vi "Memory.Pointer.Read.vi"(8 "error in (no error)":errorcluster, 9 "offset (0)":u64 format="%d bytes", 10 "length (-1: all)":i64=-1 format="%d bytes", 11 "Pointer in":refnum<class "Memory.Pointer.lvclass">) -> (0 "error out":errorcluster, 2 "data":string, 3 "Pointer out":refnum<class "Memory.Pointer.lvclass">)   [LabVIEW 2016, in "LabVIEW Memory Manager.lvlib" / "Memory.Pointer.lvclass"]
uses:
  Memory.Pointer.lvclass
  Memory.Pointer.lvclass/Memory.Pointer.ctl
  Accessors/Memory.Pointer.Get Address.vi
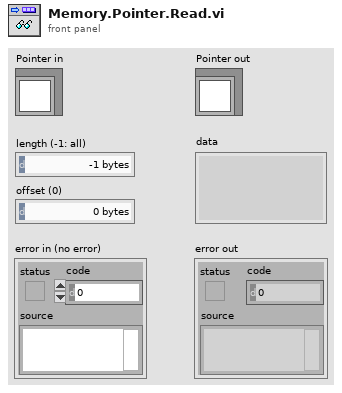
[diagram p1: front panel]
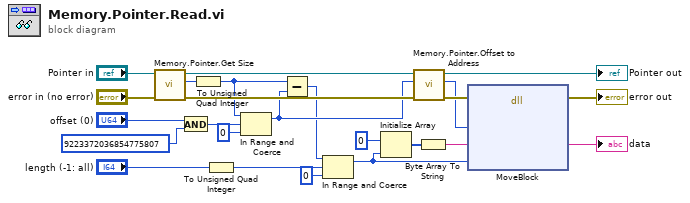
[diagram p0: block diagram]
diagram:
  n1 = call "Memory.Pointer.Get Size.vi"("error in (no error)"="error in (no error)", "Pointer in"="Pointer in") -> ("error out"=w18:errorcluster, "size"=w9:i64, "Pointer out"=w19:refnum<class "Memory.Pointer.lvclass">)  [unwired: 7 in]
  n2 = And(x="offset (0)", y=u64 9223372036854775807) -> (x .and. y?=w6:u64)
  n3 = To Unsigned Quad Integer(1:w9) -> (0:w5:u64)
  n4 = To Unsigned Quad Integer(1:"length (-1: all)") -> (0:w1:u64)
  n5 = In Range and Coerce(upper limit=w5, x=w6, lower limit=u64 0) -> (coerced(x)=w3:u64)  [unwired: 1 out]
  n6 = Subtract(x=w5, y=w3) -> (x-y=w2:u64)
  n7 = In Range and Coerce(upper limit=w2, x=w1, lower limit=u64 0) -> (coerced(x)=w17:u64)  [unwired: 1 out]
  n8 = Initialize Array(u8 0 ("element"), w17) -> (w14:u8[])
  n9 = call "Memory.Pointer.Offset to Address.vi"("error in (no error)"=w18, "offset"=w3, "Pointer in"=w19) -> ("error out"=w12:errorcluster, "offset address"=w11:u64, "Pointer out"=→"Pointer out":refnum<class "Memory.Pointer.lvclass">)  [unwired: 6 in]
  n10 = Byte Array To String(unsigned byte array=w14) -> (string=w13:string)
  n11 = dll-call lib="LabVIEW" fn="MoveBlock"(error in=w12, "src pointer"=w11, "dst pointer"=w13, "size"=w17) -> (error out=→"error out":errorcluster, "dst pointer"=→"data":string)  [unwired: 5 in, 1 out]
